vi "Actor Core.vi"(8 "error in":errorcluster, 11 "Trace Grabber Application in":refnum<class "User Interface.lvclass">) -> (0 "error out":errorcluster, 3 "Actor out":refnum<class "Actor.lvclass">)   [LabVIEW 2016, in "User Interface.lvlib" / "User Interface.lvclass"]
doc: "(<B>Filename</B>: Actor Framework.lvlib:Actor.lvclass:Actor Core.vi)\n\nReceives messages to the actor, reacts to them, and initiates any error handling that may shut the actor down.\n\nDescendant classes may override this VI to append parallel tasks for the actor to complete while it handles messages. Overrides use the Call Parent Method node."
uses:
  User Interface.lvclass
  C:/Program Files (x86)/National Instruments/LabVIEW 2016/vi.lib/ActorFramework/Actor/Actor.lvclass
  <vilib>/ActorFramework/Actor/Actor.lvclass
  <vilib>/ActorFramework/Actor/Actor.lvclass/Actor.ctl
  <vilib>/ActorFramework/Message Enqueuer/Message Enqueuer.lvclass/Message Enqueuer.ctl
  <vilib>/ActorFramework/Stop Msg/Stop Msg.lvclass/Stop Msg.ctl
  User Interface Messages/Change Delay Method Msg/Change Delay Method Msg.lvclass/Change Delay Method Msg.ctl
  User Interface Messages/Update Duration per Period Msg/Update Duration per Period Msg.lvclass/Update Duration per Period Msg.ctl
  User Interface Messages/Update Total Duration Msg/Update Total Duration Msg.lvclass/Update Total Duration Msg.ctl
  <vilib>/ActorFramework/Message Enqueuer/Init from Existing Queue.vi
  <vilib>/ActorFramework/Message Enqueuer/Enqueue Critical.vi
  <vilib>/ActorFramework/Message Enqueuer/Enqueue.vi
  <vilib>/ActorFramework/Stop Msg/Stop Msg.lvclass
  C:/Program Files (x86)/National Instruments/LabVIEW 2016/vi.lib/ActorFramework/Message/Message.lvclass
  User Interface Messages/Change Delay Method Msg/Change Delay Method Msg.lvclass
  User Interface Messages/Update Duration per Period Msg/Update Duration per Period Msg.lvclass
  User Interface Messages/Update Total Duration Msg/Update Total Duration Msg.lvclass
  <vilib>/ActorFramework/Message Priority Queue/Priority Enqueue.vi
  <vilib>/ActorFramework/Message Enqueuer/Message Enqueuer.lvclass
panel:
  out "Duration per Period":dbl format="%#_g ms"
  in  "Absolute Delay Parameters":T1 {"Absolute Delay" format="%d ps"}
  in  "Periodic Delay Parameters":cluster{"Range":i32, "Offset":i32}={"Range"=10, "Offset"=0} {"Offset" format="%d ps"; "Range" min=10 max=150 step=1 format="%d ps"}
  in  "Save Results":bool
  in  "Abort":bool
  in  "Start":bool
  in  "Free Run":bool
  in  "# Repeats":u16=20 min=1
  out "Total Duration":dbl format="%#_g ms"
  in  "# Samples per Period":u16=100 min=100 max=1000
  in  "Counting Gates":u16(ring)=500 items=["100 us"=100, "200 us"=200, "500 us"=500, "1 ms"=1000, "2 ms"=2000, "5 ms"=5000, "10 ms"=10000]
  in  "Delay Method":bool
  out "Traces":u32[](graph)
  in  "Quit":bool
  in  "Hardware Settings":bool
  # "Delay Line"
  # "Photon Counter"
  # "Measurements"
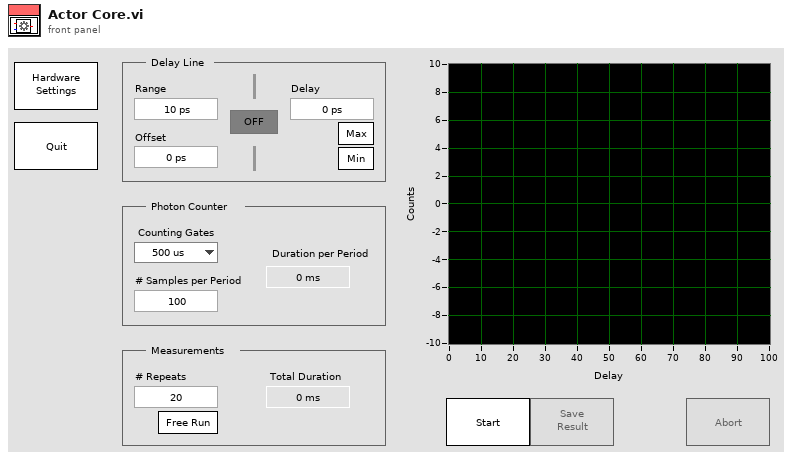
[diagram p1: front panel]
types:
  T1 = cluster{"Absolute Delay":i32, "To Min":bool, "To Max":bool}
  T2 = cluster{"Start":refnum<vi>, "Save Results":refnum<vi>, "Abort":refnum<vi>, "Hardware Settings":refnum<vi>}
  T3 = cluster{"# Samples per Period":refnum<vi>, "# Repeats":refnum<vi>, "Free Run":refnum<vi>, "Total Duration":refnum<vi>}
  T4 = enum8{"Enabled", "Disabled", "Disabled and Grayed Out"}
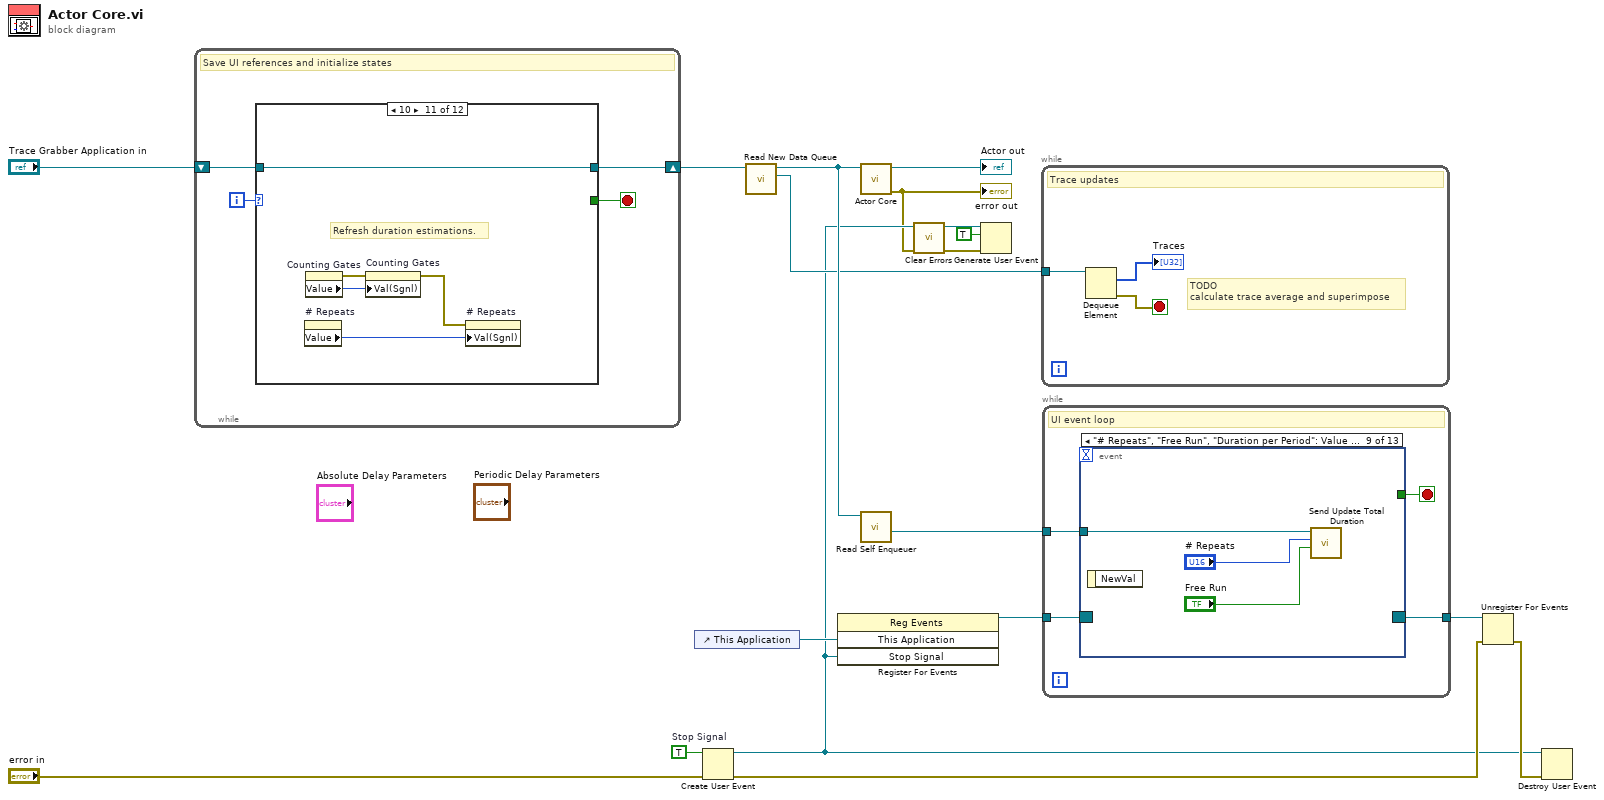
[diagram p0: block diagram]
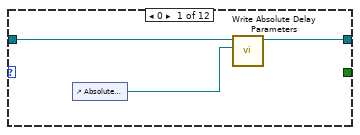
[diagram p2: hidden frame]
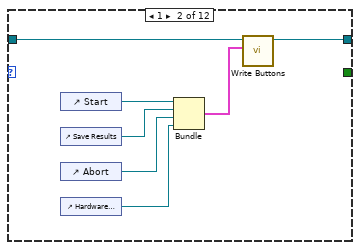
[diagram p3: hidden frame]
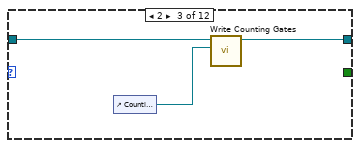
[diagram p4: hidden frame]
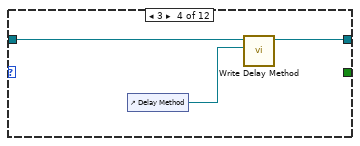
[diagram p5: hidden frame]
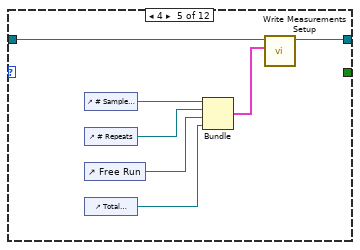
[diagram p6: hidden frame]
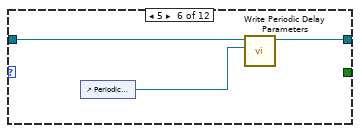
[diagram p7: hidden frame]
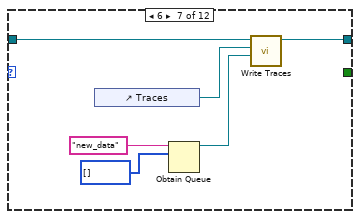
[diagram p8: hidden frame]
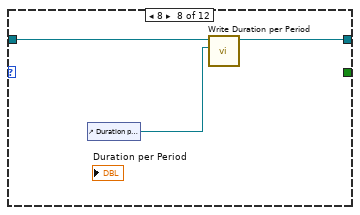
[diagram p9: hidden frame]
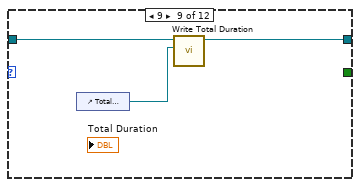
[diagram p10: hidden frame]
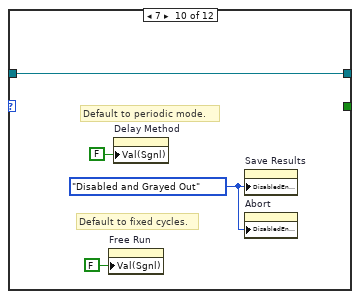
[diagram p11: hidden frame]
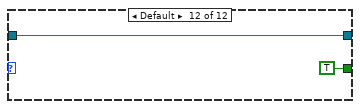
[diagram p12: hidden frame]
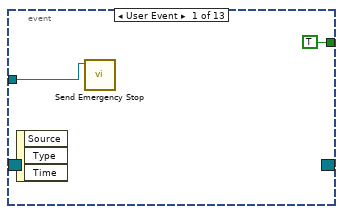
[diagram p13: hidden frame]
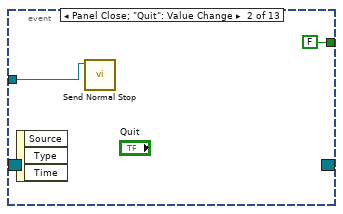
[diagram p14: hidden frame]
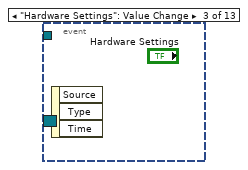
[diagram p15: hidden frame]
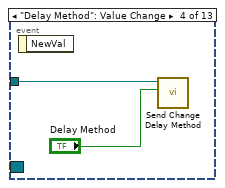
[diagram p16: hidden frame]
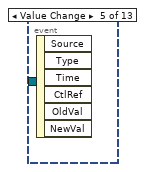
[diagram p17: hidden frame]
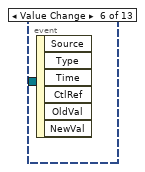
[diagram p18: hidden frame]
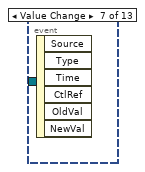
[diagram p19: hidden frame]
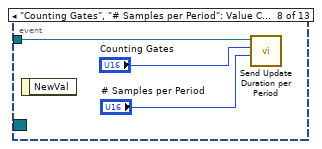
[diagram p20: hidden frame]
diagram:
  w16 = TRUE  # Stop Signal
  n1 = while {
    shift-right: [w19] -> w8
    shift-left: "Trace Grabber Application in" -> [w21]
    i -> [w20]
    stop <- w18 stop-if-true
    # "Save UI references and initialize states"
    n2 = case shown="10" w20 {
      tunnel: w21 -> [w24 w26 w32 w35 w38 w47 w51 w56 w58 w63 w68 w70]
      tunnel: [w23 w25 w33 w36 w39 w46 w52 w55 w59 w63 w68 w70] -> w19
      tunnel: [_ _ _ _ _ _ _ _ _ _ _ TRUE] -> w18
      frame 0 {
        n3 = control-ref of="Absolute Delay Parameters"() -> (w22:refnum<vi>)
        n4 = call-dynamic "Write Absolute Delay Parameters.vi"("Absolute Delay Parameters"=w22, "User Interface in"=w24) -> ("User Interface out"=w23:refnum<class "User Interface.lvclass">)  [unwired: 9 in]
      }
      frame 1 {
        n5 = control-ref of="Start"() -> (w27:refnum<vi>)
        n6 = control-ref of="Save Results"() -> (w28:refnum<vi>)
        n7 = control-ref of="Abort"() -> (w29:refnum<vi>)
        n8 = control-ref of="Hardware Settings"() -> (w30:refnum<vi>)
        n9 = Bundle("Start"=w27, "Save Results"=w28, "Abort"=w29, "Hardware Settings"=w30) -> (w31:T2)  [unwired: 1 in]
        n10 = call-dynamic "Write Buttons.vi"("Buttons"=w31, "User Interface in"=w26) -> ("User Interface out"=w25:refnum<class "User Interface.lvclass">)  [unwired: 9 in]
      }
      frame 2 {
        n11 = control-ref of="Counting Gates"() -> (w34:refnum<vi>)
        n12 = call-dynamic "Write Counting Gates.vi"("Counting Gates"=w34, "User Interface in"=w32) -> ("User Interface out"=w33:refnum<class "User Interface.lvclass">)  [unwired: 9 in]
      }
      frame 3 {
        n13 = control-ref of="Delay Method"() -> (w37:refnum<vi>)
        n14 = call-dynamic "Write Delay Method.vi"("Delay Method"=w37, "User Interface in"=w35) -> ("User Interface out"=w36:refnum<class "User Interface.lvclass">)  [unwired: 9 in]
      }
      frame 4 {
        n15 = control-ref of="# Samples per Period"() -> (w40:refnum<vi>)
        n16 = control-ref of="# Repeats"() -> (w41:refnum<vi>)
        n17 = control-ref of="Free Run"() -> (w42:refnum<vi>)
        n18 = control-ref of="Total Duration"() -> (w43:refnum<vi>)
        n19 = Bundle("# Samples per Period"=w40, "# Repeats"=w41, "Free Run"=w42, "Total Duration"=w43) -> (w44:T3)  [unwired: 1 in]
        n20 = call-dynamic "Write Measurements Setup.vi"("Measurements Setup"=w44, "User Interface in"=w38) -> ("User Interface out"=w39:refnum<class "User Interface.lvclass">)  [unwired: 9 in]
      }
      frame 5 {
        n21 = control-ref of="Periodic Delay Parameters"() -> (w45:refnum<vi>)
        n22 = call-dynamic "Write Periodic Delay Parameters.vi"("Periodic Delay Parameters"=w45, "User Interface in"=w47) -> ("User Interface out"=w46:refnum<class "User Interface.lvclass">)  [unwired: 9 in]
      }
      frame 6 {
        n23 = control-ref of="Traces"() -> (w53:refnum<vi>)
        n24 = Obtain Queue(name (unnamed)="new_data", element data type=u32[] []) -> (queue out=w48:refnum<queue>)  [unwired: 3 in, 2 out]
        n25 = call-dynamic "Write Traces.vi"("New Data Queue"=w48, "Traces"=w53, "User Interface in"=w51) -> ("User Interface out"=w52:refnum<class "User Interface.lvclass">)  [unwired: 8 in]
      }
      frame 8 {
        n26 = control-ref of="Duration per Period"() -> (w54:refnum<vi>)
        n27 = call-dynamic "Write Duration per Period.vi"("Duration per Period"=w54, "User Interface in"=w56) -> ("User Interface out"=w55:refnum<class "User Interface.lvclass">)  [unwired: 9 in]
      }
      frame 9 {
        n28 = control-ref of="Total Duration"() -> (w57:refnum<vi>)
        n29 = call-dynamic "Write Total Duration.vi"("Total Duration"=w57, "User Interface in"=w58) -> ("User Interface out"=w59:refnum<class "User Interface.lvclass">)  [unwired: 9 in]
      }
      frame 7 {
        w60 = T4."Disabled and Grayed Out" ("Disabled")
        # "Default to fixed cycles."
        # "Default to periodic mode."
        n30 = property on="Free Run" class="Bool (strict)"("Val(Sgnl)"=FALSE ("Value (Signaling)")) -> ()  [unwired: 2 in, 2 out]
        n31 = property on="Delay Method" class="Bool (strict)"("Val(Sgnl)"=FALSE ("Value (Signaling)")) -> ()  [unwired: 2 in, 2 out]
        n32 = property on="Save Results" class="Bool"("DisabledEnum"=w60) -> ()  [unwired: 2 in, 2 out]
        n33 = property on="Abort" class="Bool"("DisabledEnum"=w60) -> ()  [unwired: 2 in, 2 out]
      }
      frame 10 {
        # "Refresh duration estimations."
        n34 = property on="# Repeats" class="DigNum (strict)"() -> ("Value"=w65:u16)  [unwired: 2 in, 2 out]
        n35 = property on="Counting Gates" class="Ring (strict)"() -> (error out=w67:errorcluster, "Value"=w66:u16)  [unwired: 2 in, 1 out]
        n36 = property on="Counting Gates" class="Ring (strict)"(error in=w67, "Val(Sgnl)"=w66) -> (error out=w64:errorcluster)  [unwired: 1 in, 1 out]
        n37 = property on="# Repeats" class="DigNum (strict)"(error in=w64, "Val(Sgnl)"=w65) -> ()  [unwired: 1 in, 2 out]
      }
      frame Default {
      }
    }
  }
  n38 = control-ref of="This Application"() -> (w14:refnum<vi>)
  n39 = Create User Event(user event datatype=w16, error in="error in") -> (user event=w3:refnum<user-event>, error out=w4:errorcluster)
  n40 = call-dynamic "Read New Data Queue.vi"("User Interface in"=w8) -> ("New Data Queue"=w6:refnum<queue>, "User Interface out"=w7:refnum<class "User Interface.lvclass">)  [unwired: 9 in]
  n41 = register-events(w14, w3) -> (reference out=w13:refnum<event-registration>)  [unwired: 2 in, 1 out]
  n42 = call-parent "Actor Core.vi"("Actor in"=w7) -> ("error out"=w1:errorcluster, "Actor out"=→"Actor out":refnum<class "Actor.lvclass">)  [unwired: 9 in]
  "error out" <- w1
  n43 = call <vilib>:"Read Self Enqueuer.vi"("Actor"=w7) -> ("Self Enqueuer"=w10:refnum<class "Message Enqueuer.lvclass">)  [unwired: 10 in]
  n44 = call <vilib>:"Clear Errors.vi"("error in (no error)"=w1) -> ("error out"=w2:errorcluster)  [unwired: 5 in, 1 out]
  n45 = Generate User Event(user event=w3, event data cluster=TRUE ("event data"), error in=w2) -> ()  [unwired: 1 in, 2 out]
  n46 = while {
    tunnel: w6 -> [w73]
    stop <- w71 stop-if-true
    # "TODO\ncalculate trace average and superimpose"
    # "Trace updates"
    n47 = Dequeue Element(queue=w73) -> (element=→"Traces":u32[], error out=w71:errorcluster)  [unwired: 2 in, 2 out]
  }
  n48 = while {
    tunnel: w13 -> [w77]
    tunnel: [w75] -> w12
    tunnel: w10 -> [w74]
    stop <- w76 stop-if-true
    # "UI event loop"
    n49 = event shown="[8] \"# Repeats\", \"Free Run\", \"Duration per Period\": Value Change" {
      selector: w77 -> [_ _ _ _ _ _ _ _ _ _ _ _ _]
      dyn-events: [_ _ _ _ _ _ _ _ _ _ _ _ _] -> w75
      timeout: _ -> [_ _ _ _ _ _ _ _ _ _ _ _ _]
      tunnel: [TRUE FALSE _ _ _ _ _ _ _ _ _ _ FALSE] -> w76
      tunnel: w74 -> [w78 w80 _ w83 _ _ _ w86 w89 _ _ _ _]
      event User Event {
        n50 = event-data() -> ()  [unwired: 1 in, 3 out]
        n51 = call <vilib>:"Send Emergency Stop.vi"("Message Enqueuer"=w78) -> ()  [unwired: 10 in, 1 out]
      }
      event Panel Close; "Quit": Value Change {
        n52 = event-data() -> ()  [unwired: 1 in, 3 out]
        n53 = call <vilib>:"Send Normal Stop.vi"("Message Enqueuer"=w80) -> ()  [unwired: 10 in, 1 out]
      }
      event "Hardware Settings": Value Change {
        n54 = event-data() -> ()  [unwired: 1 in, 3 out]
      }
      event "Delay Method": Value Change {
        n55 = event-data() -> ()  [unwired: 1 in, 1 out]
        n56 = call "Send Change Delay Method.vi"("Is absolute delay mode?"="Delay Method", "Message Enqueuer"=w83) -> ()  [unwired: 8 in, 2 out]
      }
      event "Periodic Delay Parameters.Range", "Periodic Delay Parameters.Offset": Value Change {
        n57 = event-data() -> ()  [unwired: 1 in, 6 out]
      }
      event "Absolute Delay Parameters.Absolute Delay": Value Change {
        n58 = event-data() -> ()  [unwired: 1 in, 6 out]
      }
      event "Absolute Delay Parameters.To Max", "Absolute Delay Parameters.To Min": Value Change {
        n59 = event-data() -> ()  [unwired: 1 in, 6 out]
      }
      event "Counting Gates", "# Samples per Period": Value Change {
        n60 = event-data() -> ()  [unwired: 1 in, 1 out]
        n61 = call "Send Update Duration per Period.vi"("# Samples per Period"="# Samples per Period", "Counting Gates"="Counting Gates", "Message Enqueuer"=w86) -> ()  [unwired: 7 in, 2 out]
      }
      event "# Repeats", "Free Run", "Duration per Period": Value Change {
        n62 = event-data() -> ()  [unwired: 1 in, 1 out]
        n63 = call "Send Update Total Duration.vi"("Free Run?"="Free Run", "# Repeats"="# Repeats", "Message Enqueuer"=w89) -> ()  [unwired: 7 in, 2 out]
      }
      event "Start": Value Change {
        n64 = event-data() -> ()  [unwired: 1 in, 6 out]
      }
      event "Abort": Value Change {
        n65 = event-data() -> ()  [unwired: 1 in, 6 out]
      }
      event "Save Results": Value Change {
        n66 = event-data() -> ()  [unwired: 1 in, 6 out]
      }
      event Application Instance Close {
        n67 = event-data() -> ()  [unwired: 1 in, 3 out]
      }
    }
  }
  n68 = Unregister For Events(event registration refnum=w12, error in=w4) -> (error out=w11:errorcluster)
  n69 = Destroy User Event(user event=w3, error in=w11) -> ()  [unwired: 1 out]
